vi "Init HTTP Server.vi"(8 "error in (no error)":errorcluster, 11 "VMR Server in":refnum<class "VMR Server.lvclass">) -> (0 "error out":errorcluster, 3 "VMR Server out":refnum<class "VMR Server.lvclass">)   [LabVIEW 2022 SP3, in "VMR Server.lvlib" / "VMR Server.lvclass"]
uses:
  VMR Server.lvclass
  VMR Server.lvclass/VMR Server.ctl
  VMR Actor API/VMR Actor API.lvclass
  C:/Program Files (x86)/National Instruments/LabVIEW 2022/vi.lib/IlluminatedG/IG HTTP Server/HTTP Server/Service/Service.lvclass
  <vilib>/IlluminatedG/IG HTTP Server/HTTP Server/Server/Server.lvclass
  AudioSummaryController/AudioSummaryController.lvclass
  C:/dev/lv/2022/touchcontrol/VMR Server/VMR Actor API/VMR Actor API.lvclass
  C:/Program Files (x86)/National Instruments/LabVIEW 2022/resource/AFDebug/Protected Actor Handle/Protected Actor Handle.lvclass
  C:/Program Files (x86)/National Instruments/LabVIEW 2022/vi.lib/IlluminatedG/IG HTTP Server/HTTP Server/Controller/Controller.lvclass
  C:/Program Files (x86)/National Instruments/LabVIEW 2022/vi.lib/IlluminatedG/IG HTTP Server/HTTP Server/Handler/Handler.lvclass
  C:/dev/lv/2022/touchcontrol/VMR Server/AudioSummaryController/AudioSummaryController.lvclass
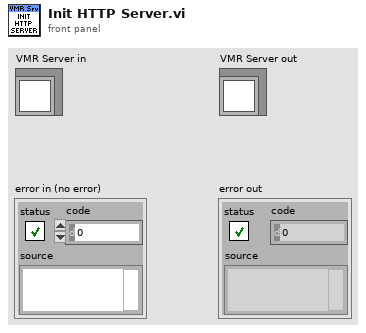
[diagram p1: front panel]
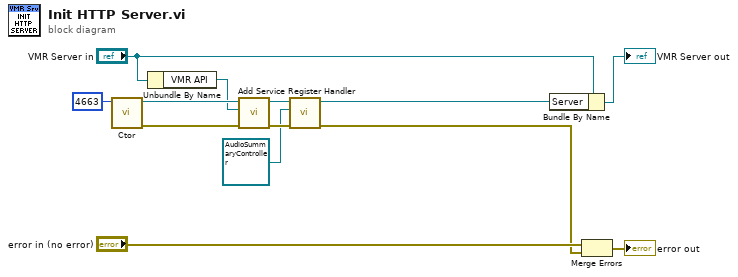
[diagram p0: block diagram]
diagram:
  n1 = call <vilib>:"Ctor.vi"("HTTP Port (80)"=u16 4663) -> ("error out"=w7:errorcluster, "Server out"=w10:refnum<class "Server.lvclass">)  [unwired: 9 in]
  n2 = Unbundle By Name("VMR Server in") -> ("VMR API"=w9:refnum<class "VMR Actor API.lvclass">)
  n3 = call <vilib>:"Add Service.vi"("error in (no error)"=w7, "Service"=w9, "Server in"=w10) -> ("error out"=w5:errorcluster, "Server out"=w3:refnum<class "Server.lvclass">)  [unwired: 7 in]
  n4 = call <vilib>:"Register Handler.vi"("error in (no error)"=w5, "Handler"=refnum<class "AudioSummaryController.lvclass"> refnum ("VMR Server.lvlib:AudioSummaryController.lvclass"), "Server in"=w3) -> ("error out"=w4:errorcluster, "Server in"=w2:refnum<class "Server.lvclass">)  [unwired: 7 in]
  n5 = Bundle By Name(cluster="VMR Server in", "Server"=w2) -> (→"VMR Server out":refnum<class "VMR Server.lvclass">)
  n6 = Merge Errors("error in (no error)", w4) -> (→"error out":errorcluster)
